vi "New timing.vi"(8 "error in":errorcluster, 11 "core timeing configuration (default)":T1={"driftMax"=425000000, "delayComp"=0, "irigControlVal"=[0, 0, 0, 0], "irigYears"=2000, "irigType"=1, "jumpThreshPPT"=425000000, "jumpThreshNS"=200000, "timerRollover"=0, "timeSourceSelect"=0, "timeSyncSelect"=0, "timeEnableUserInputThresh"=FALSE, "timeInputThreshVal"=[0, 0], "driftSyncSelect"=0, "driftEnableUserInputThresh"=FALSE, "driftInputThreshVal"=[0, 0], "resolution"=0, "timerValue"=0} {"resolution" items=["Item1NS", "Item1US"]; "driftSyncSelect" items=["None", "PPS0", "PPS1", "PWMIRIG0", "PWMIRIG1", "AMIRIG", "Item10MHZ", "HOST"]; "timeSyncSelect" items=["None", "PPS0", "PPS1", "PWMIRIG0", "PWMIRIG1", "AMIRIG"]; "timeSourceSelect" items=["None", "PPS0", "PPS1", "PWMIRIG0", "PWMIRIG1", "AMIRIG", "Item10MHZ"]; "irigType" items=["A", "B"]}) -> (0 "error out":errorcluster, 3 "new timing out":refnum<k24>)   [LabVIEW 2020, in "Ballard_1553_Hardware_ni.lvlib"]
uses:
  Ballard_1553_Hardware_ni.lvlib
  C:/Users/Administrator/Desktop/GIT/Ballard-MIL-STD-1553-Custom-Device/Source/System Explorer/SubVIs/Parse XML Ballard/1.2/BTIXML_SerDes.dll
  Ballard-MIL-STD-1553-Custom-Device/Source/System Explorer/SubVIs/Parse XML Ballard/1.2/BTIXML_SerDes.dll
  _typedefs/core_timing_type.ctl
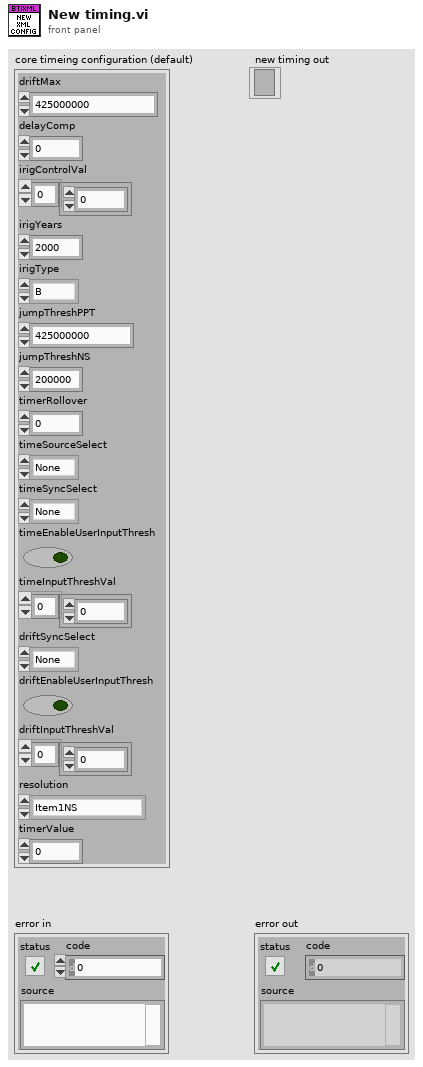
[diagram p1: front panel]
types:
  T1 = typedef "Ballard_1553_Hardware_ni.lvlib/core_timing_type.ctl" = cluster{"driftMax":u32, "delayComp":i32, "irigControlVal":u8[], "irigYears":u32, "irigType":i32, "jumpThreshPPT":u32, "jumpThreshNS":u32, "timerRollover":u64, "timeSourceSelect":i32, "timeSyncSelect":i32, "timeEnableUserInputThresh":bool, "timeInputThreshVal":u8[], "driftSyncSelect":i32, "driftEnableUserInputThresh":bool, "driftInputThreshVal":u8[], "resolution":i32, "timerValue":u64}
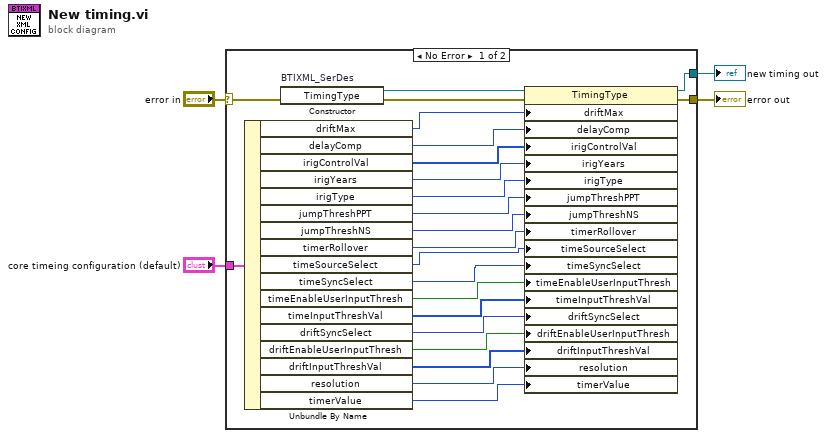
[diagram p0: block diagram]
diagram:
  n1 = case shown="No Error" "error in" {
    selector: "error in" -> [w27 w28]
    tunnel: [w24 w28] -> w3
    tunnel: [w23 _] -> w2
    tunnel: "core timeing configuration (default)" -> [w22 _]
    frame No Error {
      n2 = Unbundle By Name(w22) -> ("driftMax"=w21:u32, "delayComp"=w20:i32, "irigControlVal"=w19:u8[], "irigYears"=w18:u32, "irigType"=w17:i32, "jumpThreshPPT"=w16:u32, "jumpThreshNS"=w15:u32, "timerRollover"=w14:u64, "timeSourceSelect"=w13:i32, "timeSyncSelect"=w12:i32, "timeEnableUserInputThresh"=w11:bool, "timeInputThreshVal"=w10:u8[], "driftSyncSelect"=w9:i32, "driftEnableUserInputThresh"=w8:bool, "driftInputThreshVal"=w7:u8[], "resolution"=w6:i32, "timerValue"=w5:u64)
      n3 = constructor on="BTIXML_SerDes" class="TimingType"(error in=w27) -> (reference out=w26:refnum<k24>, error out=w25:errorcluster)  [unwired: 2 in, 1 out]
      n4 = property class="TimingType"(reference=w26, error in=w25, "driftMax"=w21, "delayComp"=w20, "irigControlVal"=w19, "irigYears"=w18, "irigType"=w17, "jumpThreshPPT"=w16, "jumpThreshNS"=w15, "timerRollover"=w14, "timeSourceSelect"=w13, "timeSyncSelect"=w12, "timeEnableUserInputThresh"=w11, "timeInputThreshVal"=w10, "driftSyncSelect"=w9, "driftEnableUserInputThresh"=w8, "driftInputThreshVal"=w7, "resolution"=w6, "timerValue"=w5) -> (reference out=w23:refnum<k24>, error out=w24:errorcluster)
    }
    frame Error {
    }
  }
  "error out" <- w3
  "new timing out" <- w2
